vi "Objective Align.vi"() -> ()   [LabVIEW 2021]
uses:
  Objective Align Controls/Objective Align Notifier Type Def.ctl
  Objective Align Controls/Objective Align Actions.ctl
  <vilib>/vision/Image Controls.llb/IMAQ Image.ctl
  Hardware Configuration/Hardware Configuration Controls/Device Type.ctl
  Hardware Configuration/Hardware Configuration Controls/Device Function.ctl
  Device Library/Stages/Stages Controls/Stage Actions.ctl
panel:
  out "Top Z shift":dbl
  out "Bottom Z shift":dbl
  in  "Sample Z factor":dbl
  in  "Obj. Z factor":dbl
  in  "Quit":bool
  in  "Frame Accumulation":u16
  in  "CCD offset":dbl
  out "XY shift":dbl[](array[numeric])
  out "Coord":i32[][](array[numeric])
  out "Z metric":dbl[](array[numeric])
  out "ROI stack":u16[][][](array[numeric])
  in  "ROI Size":i32
  in  "XY Step Size (µm)":dbl
  in  "Pixel Size (µm)":dbl
  in  "Start Align":bool
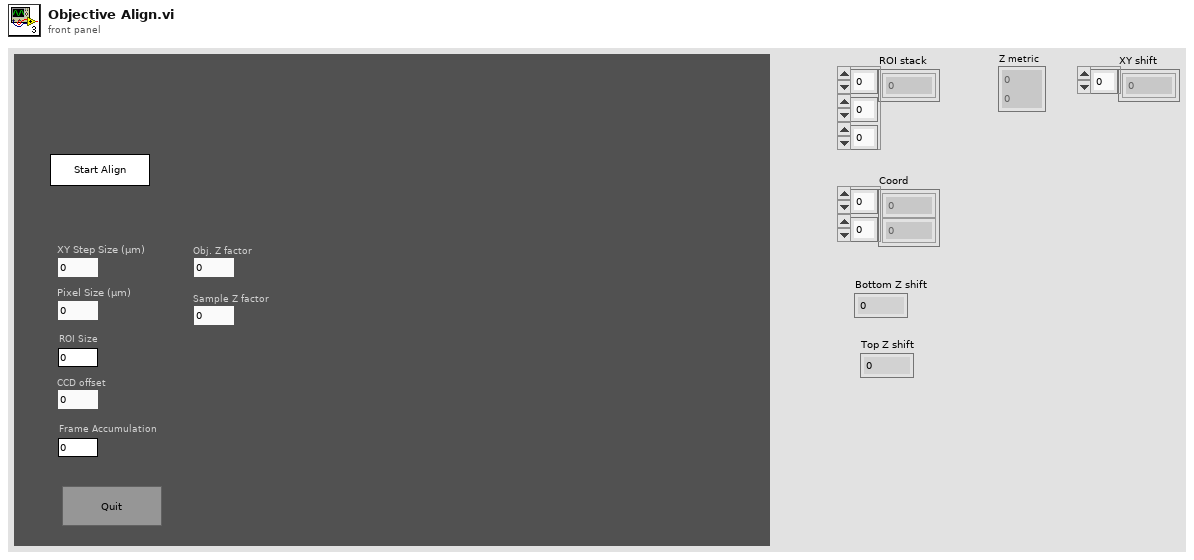
[diagram p1: front panel]
types:
  T1 = typedef "IMAQ Image.ctl" = refnum<image>
  T2 = typedef "Objective Align Actions.ctl" = enum16{"idle", "Start Align", "Move Z stage", "Move XY Stage", "Get Image", "Get Position", "Exit", "Quit"}
  T3 = typedef "Objective Align Notifier Type Def.ctl" = cluster{"Action":T2, "Pixel Size (µm)":dbl, "XY Step Size (µm)":dbl, "Image Ref":T1, "ROI Size":i32, "ROI Stack":u16[][][], "Frame Accumulation":u16, "CCD offset":dbl, "obj. Z factor":dbl, "sample Z factor ":dbl}
  T4 = typedef "Device Function.ctl" = enum16{"Primary", "Secondary", "Overview", "Wide Field Drift Correction", "642 nm Excitation", "560 nm Excitation", "940 nm Excitation", "546 nm Excitation", "488 nm Excitation", "405 nm Excitation", "Objective Drift Correction", "4Pi Focus Lock", "4Pi Objective Lock", "Objective XY", "Objective Z", "Sample XY", "Sample Coarse Z", "Sample Z", "4Pi Lower", "4Pi Upper", "Em Small", "Em Large", "Ex Small", "Ex Large", "Mojo", "Adj Cavity", "Line Scanning", "Alert"}
  T5 = typedef "Device Type.ctl" = enum16{"AOTF", "Camera", "Deformable Mirror", "Laser", "Flip Mirror", "Shutter", "Stage", "Waveform", "FPGA", "Email"}
  T6 = typedef "Stage Actions.ctl" = enum16{"Get Position", "SERVO OFF", "SERVO ON", "SERVO ON/OFF", "MVR", "MOVE", "HALT", "ONTARGET", "ERROR", "REFERENCE", "INIT", "VELOCITY", "STATUS", "EXIT", "HOME", "ZEROPOS", "NANOPOS", "ANALOG", "QUIT"}
  T7 = typedef "4Pi OBJ Lock-2D Gaussian - Best Fit Parameters.ctl" = cluster{"Amplitude":dbl, "X Position":dbl, "Y Position":dbl, "X Width":dbl, "Y Width":dbl, "Offset":dbl}
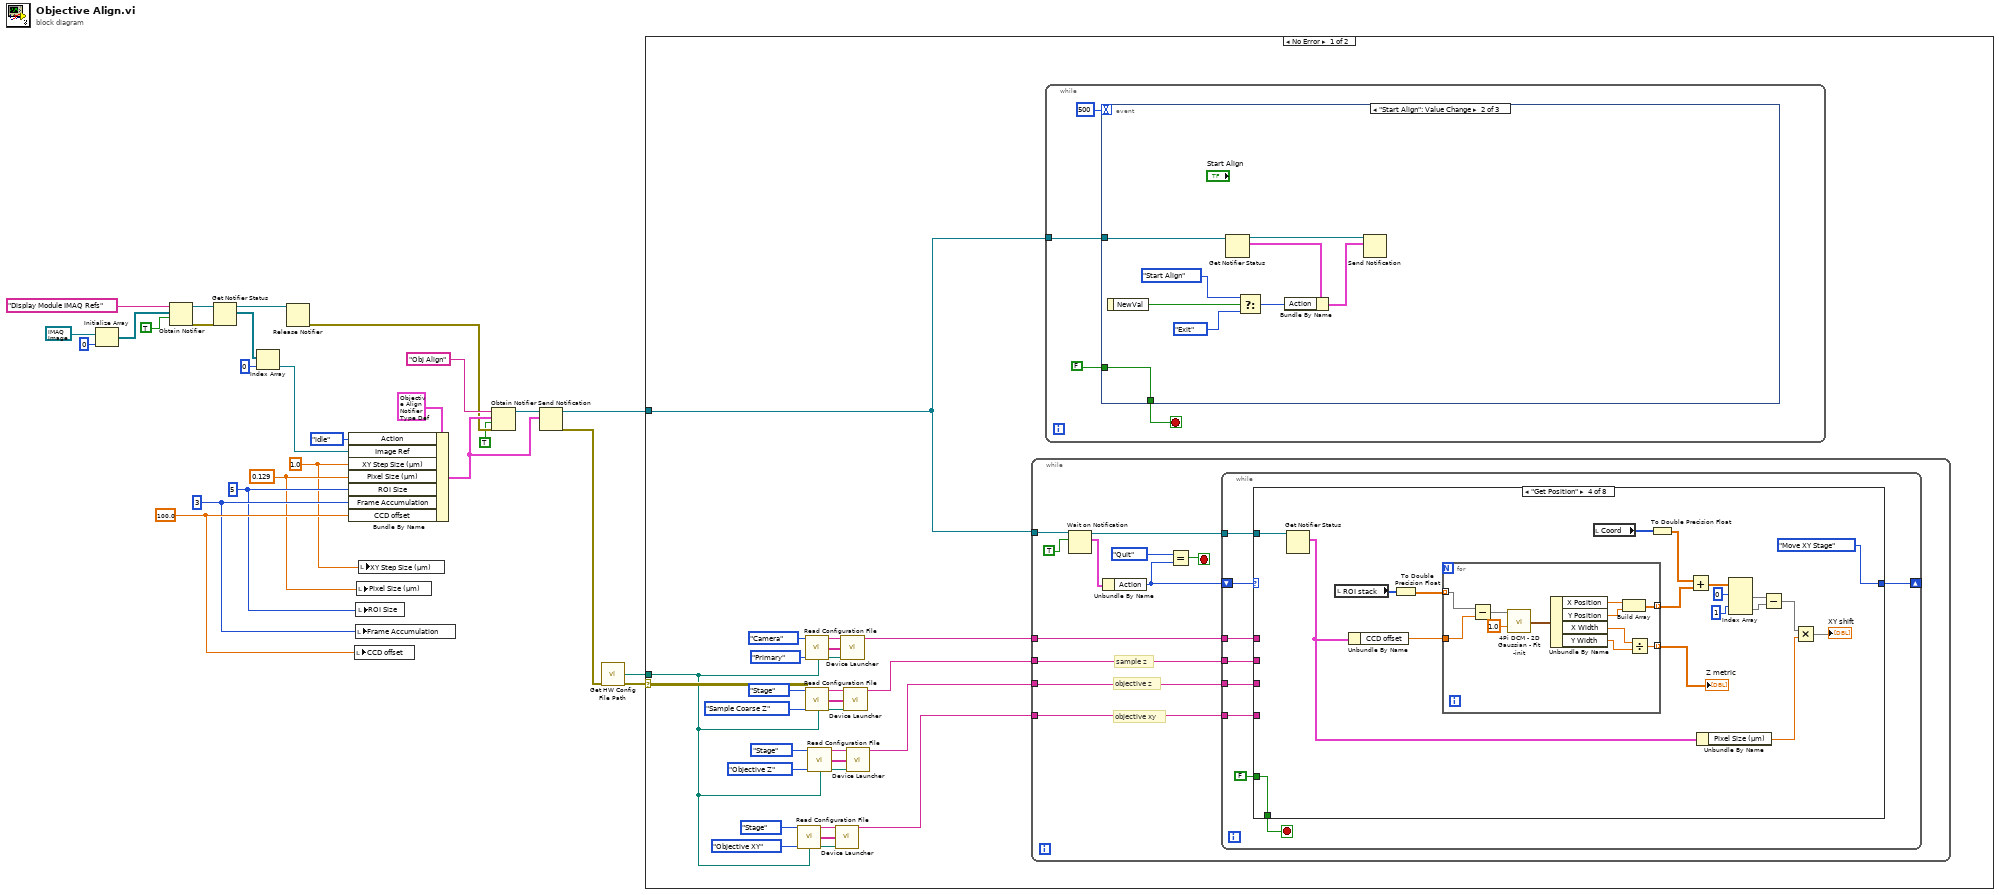
[diagram p0: block diagram]
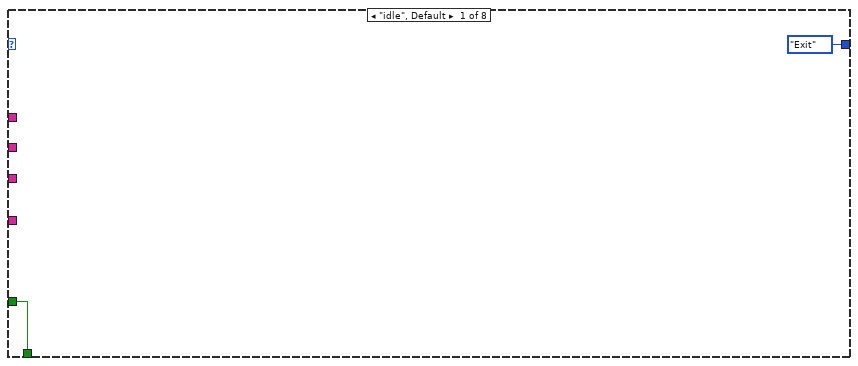
[diagram p2: hidden frame]
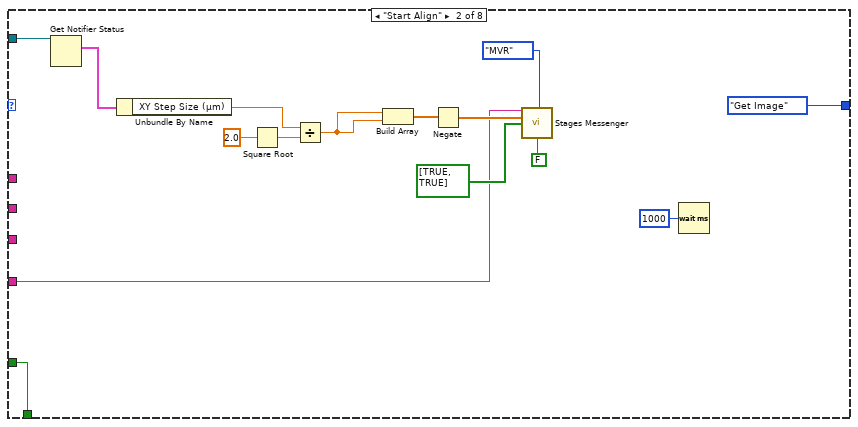
[diagram p3: hidden frame]
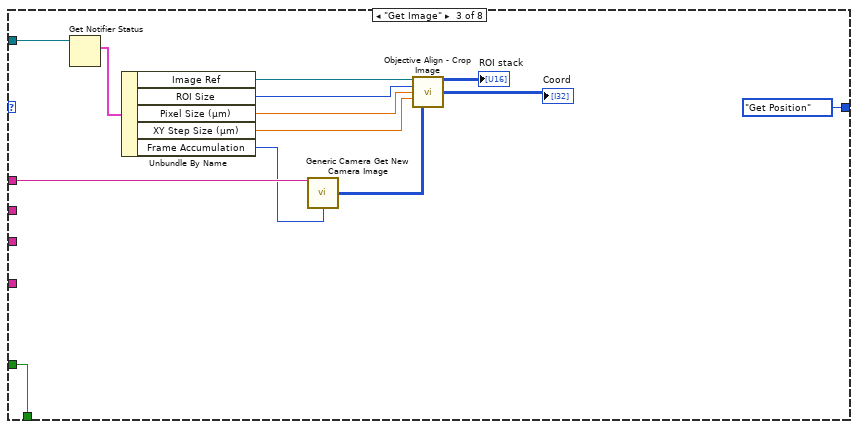
[diagram p4: hidden frame]
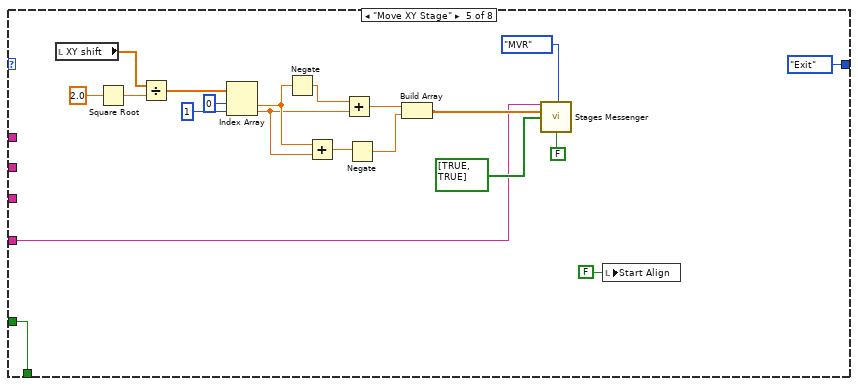
[diagram p5: hidden frame]
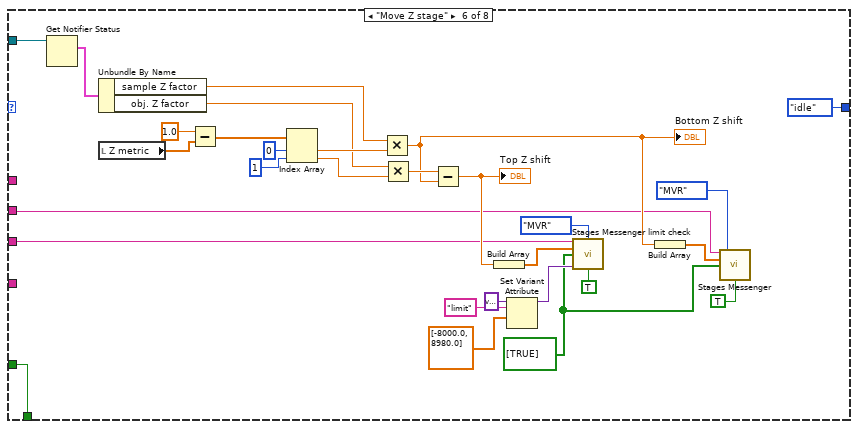
[diagram p6: hidden frame]
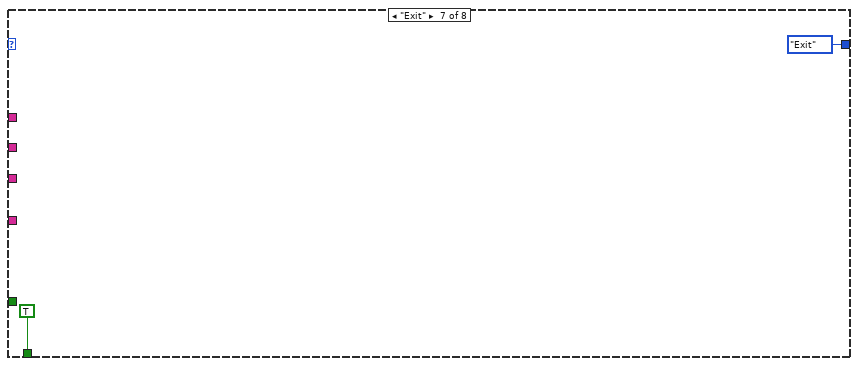
[diagram p7: hidden frame]
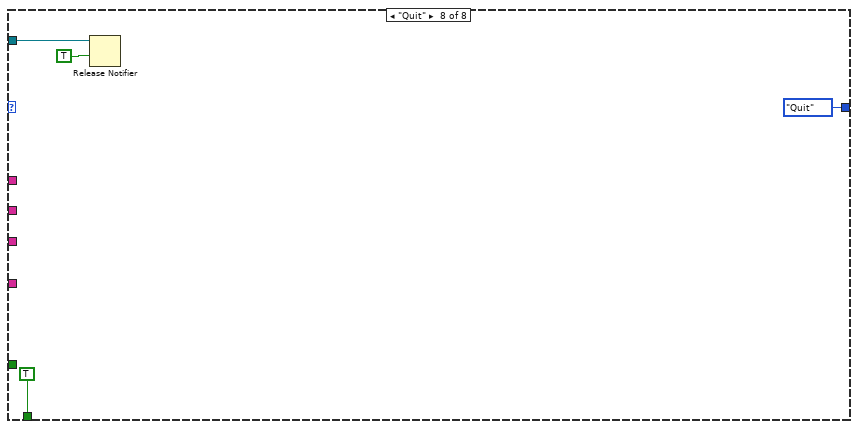
[diagram p8: hidden frame]
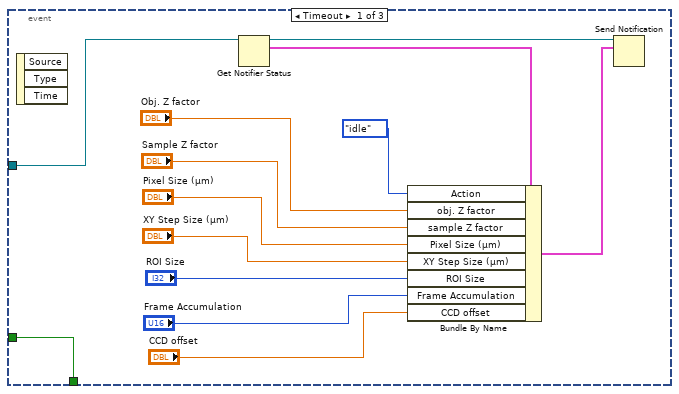
[diagram p9: hidden frame]
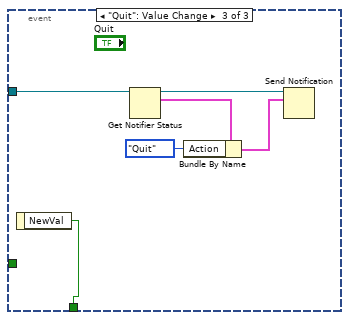
[diagram p10: hidden frame]
diagram:
  w8 = 100.0 ("CCD offset")
  w7 = u16 3 ("Frame Accumulation")
  w6 = 5 ("ROI Size")
  w5 = 0.129 ("Pixel Size (µm)")
  w4 = 1.0 ("XY Step Size (µm)")
  n1 = Initialize Array(T1 refnum ("New Image"), 0 ("dimension size")) -> (w21:T1[])
  n2 = Obtain Notifier(name (unnamed)="Display Module IMAQ Refs", notification data type=w21, create if not found? (T)=TRUE) -> (notifier out=w20:refnum<notifier>, error out=w19:errorcluster)  [unwired: 1 in, 1 out]
  n3 = Get Notifier Status(notifier=w20, error in (no error)=w19) -> (notifier out=w3:refnum<notifier>, current notification=w18:T1[])  [unwired: 3 out]
  n4 = Index Array(array=w18, index=0) -> (element=w16:T1)
  n5 = Release Notifier(notifier=w3) -> (error out=w2:errorcluster)  [unwired: 2 in, 2 out]
  n6 = Bundle By Name(cluster=T3 {"Action"=enum."Start Align", "Pixel Size (µm)"=0.0, "XY Step Size (µm)"=0.0, "Image Ref"=refnum, "ROI Size"=0, "ROI Stack"=[], "Frame Accumulation"=0, "CCD offset"=0.0, "obj. Z factor"=0.0, "sample Z factor "=0.0} ("Objective Align Notifier Type"), "Action"=Objective_Align_Actions."idle", "Image Ref"=w16, "XY Step Size (µm)"=w4, "Pixel Size (µm)"=w5, "ROI Size"=w6, "Frame Accumulation"=w7, "CCD offset"=w8) -> (w13:T3)
  n7 = local write "CCD offset"(w8) -> ()
  n8 = local write "Frame Accumulation"(w7) -> ()
  n9 = local write "ROI Size"(w6) -> ()
  n10 = local write "Pixel Size (µm)"(w5) -> ()
  n11 = local write "XY Step Size (µm)"(w4) -> ()
  n12 = Obtain Notifier(name (unnamed)="Obj Align", notification data type=w13, create if not found? (T)=TRUE, error in (no error)=w2) -> (notifier out=w14:refnum<notifier>)  [unwired: 2 out]
  n13 = Send Notification(notification=w13, notifier=w14) -> (notifier out=w9:refnum<notifier>, error out=w12:errorcluster)  [unwired: 1 in]
  n14 = call "Get HW Config File Path.vi"("Error"=w12) -> ("File Path"=w10:path, "Error"=w11:errorcluster)  [unwired: 13 in]
  n15 = case shown="No Error" w11 {
    tunnel: w9 -> [w43 _]
    tunnel: w10 -> [w29 _]
    frame No Error {
      n16 = call "Read Configuration File.vi"("Device Type"=Device_Type."Stage", "Device Function"=Device_Function."Objective XY", "Config File Path"=w29) -> ("Unique Notifier Name"=w48:string, "Device Ports/IDs/Channels"=w47:string[], "Device Engine Path"=w46:path)  [unwired: 9 in, 1 out]
      n17 = call "Read Configuration File.vi"("Device Type"=Device_Type."Camera", "Device Function"=Device_Function."Primary", "Config File Path"=w29) -> ("Unique Notifier Name"=w53:string, "Device Ports/IDs/Channels"=w51:string[], "Device Engine Path"=w52:path)  [unwired: 9 in, 1 out]
      n18 = call "Read Configuration File.vi"("Device Type"=Device_Type."Stage", "Device Function"=Device_Function."Sample Coarse Z", "Config File Path"=w29) -> ("Unique Notifier Name"=w38:string, "Device Ports/IDs/Channels"=w39:string[], "Device Engine Path"=w40:path)  [unwired: 9 in, 1 out]
      n19 = call "Read Configuration File.vi"("Device Type"=Device_Type."Stage", "Device Function"=Device_Function."Objective Z", "Config File Path"=w29) -> ("Unique Notifier Name"=w30:string, "Device Ports/IDs/Channels"=w31:string[], "Device Engine Path"=w32:path)  [unwired: 9 in, 1 out]
      n20 = call "Device Launcher.vi"("Notifier Name"=w48, "Device Ports/IDs/Channels"=w47, "Device Engine Path"=w46) -> ("Notifier Name"=w42:string)  [unwired: 11 in, 1 out]
      n21 = call "Device Launcher.vi"("Notifier Name"=w53, "Device Ports/IDs/Channels"=w51, "Device Engine Path"=w52) -> ("Notifier Name"=w41:string)  [unwired: 11 in, 1 out]
      n22 = call "Device Launcher.vi"("Notifier Name"=w38, "Device Ports/IDs/Channels"=w39, "Device Engine Path"=w40) -> ("Notifier Name"=w35:string)  [unwired: 11 in, 1 out]
      n23 = call "Device Launcher.vi"("Notifier Name"=w30, "Device Ports/IDs/Channels"=w31, "Device Engine Path"=w32) -> ("Notifier Name"=w28:string)  [unwired: 11 in, 1 out]
      n24 = while {
        tunnel: w43 -> [w62]
        tunnel: w42 -> [w57]
        tunnel: w41 -> [w56]
        tunnel: w35 -> [w55]
        tunnel: w28 -> [w54]
        stop <- w60 stop-if-true
        # "objective xy"
        # "sample z"
        # "objective z"
        n25 = Wait on Notification(notifier=w62, ignore previous (F)=TRUE) -> (notifier out=w59:refnum<notifier>, notification=w63:T3)  [unwired: 2 in, 2 out]
        n26 = Unbundle By Name(w63) -> ("Action"=w58:T2)
        n27 = Equal?(x=Objective_Align_Actions."Quit", y=w58) -> (x = y?=w60:bool)
        n28 = while {
          tunnel: w59 -> [w70]
          shift-right: [w68] -> _
          shift-left: w58 -> [w71]
          tunnel: w57 -> [w69]
          tunnel: w56 -> [w67]
          tunnel: w55 -> [w66]
          tunnel: w54 -> [w65]
          stop <- w72 stop-if-true
          n29 = case shown="\"Get Position\"" w71 {
            tunnel: FALSE -> [w74 w90 w91 w122 w135 w181 _ _]
            tunnel: [w74 w90 w91 w122 w135 w181 TRUE TRUE] -> w72
            tunnel: w70 -> [_ w89 w103 w121 _ w180 _ w187]
            tunnel: w69 -> [_ w78 _ _ w137 _ _ _]
            tunnel: [Objective_Align_Actions."Exit" ("Action") Objective_Align_Actions."Get Image" ("Action") Objective_Align_Actions."Get Position" ("Action") Objective_Align_Actions."Move XY Stage" ("Action") Objective_Align_Actions."Exit" ("Action") Objective_Align_Actions."idle" ("Action") Objective_Align_Actions."Exit" ("Action") Objective_Align_Actions."Quit" ("Action")] -> w68
            tunnel: w67 -> [_ _ w101 _ _ _ _ _]
            tunnel: w66 -> [_ _ _ _ _ w157 _ _]
            tunnel: w65 -> [_ _ _ _ _ w161 _ _]
            frame "idle", Default {
            }
            frame "Start Align" {
              n30 = Get Notifier Status(notifier=w89) -> (current notification=w88:T3)  [unwired: 1 in, 4 out]
              n31 = Unbundle By Name(w88) -> ("XY Step Size (µm)"=w85:dbl)
              n32 = Square Root(x=2.0) -> (sqrt(x)=w86:dbl)
              n33 = Divide(x=w85, y=w86) -> (x/y=w84:dbl)
              n34 = Build Array(w84, w84) -> (w83:dbl[])
              n35 = Negate(x=w83) -> (-x=w81:dbl[])
              n36 = call "Stages Messenger.vi"("Stage Notifier Name"=w78, "Actions"=Stage_Actions."MVR", "Setpoint"=w81, "Axis"=bool[] [TRUE, TRUE], "Exit While Busy?"=FALSE) -> ()  [unwired: 6 in, 5 out]
              n37 = Wait (ms)(milliseconds to wait=u32 1000) -> ()  [unwired: 1 out]
            }
            frame "Get Image" {
              n38 = Get Notifier Status(notifier=w103) -> (current notification=w102:T3)  [unwired: 1 in, 4 out]
              n39 = Unbundle By Name(w102) -> ("Image Ref"=w99:T1, "ROI Size"=w98:i32, "Pixel Size (µm)"=w97:dbl, "XY Step Size (µm)"=w96:dbl, "Frame Accumulation"=w100:u16)
              n40 = call "Generic Camera Get New Camera Image.vi"("Camera Notifier Name"=w101, "Frames"=w100) -> ("Image - U16"=w95:u16[][])  [unwired: 11 in, 2 out]
              n41 = call "Objective Align - Crop Image.vi"("Image Ref"=w99, "ROI Size"=w98, "Pixel Size (µm)"=w97, "XY Step Size (µm)"=w96, "Input Image - U16"=w95) -> ("Output Image Stack"=→"ROI stack":u16[][][], "Coord"=→"Coord":i32[][])  [unwired: 9 in]
            }
            frame "Get Position" {
              n42 = Get Notifier Status(notifier=w121) -> (current notification=w107:T3)  [unwired: 1 in, 4 out]
              n43 = local read "ROI stack"() -> (w120:u16[][][])
              n44 = Unbundle By Name(w107) -> ("CCD offset"=w118:dbl)
              n45 = To Double Precision Float(number=w120) -> (double precision float=w119:dbl[][][])
              n46 = for {
                tunnel: w119 -> [w131] mode=indexing
                tunnel: w118 -> [w130]
                tunnel: [w126] -> w117 mode=indexing
                tunnel: [w123] -> w114 mode=indexing
                n47 = Subtract(x=w131, y=w130) -> (x-y=w129:dbl[][])
                n48 = call "4Pi DCM - 2D Gaussian - Fit -init.vi"("Image In (DBL)"=w129, "width"=1.0) -> ("Best Fit Params"=w132:T7)  [unwired: 12 in, 1 out]
                n49 = Unbundle By Name(w132) -> ("X Position"=w125:dbl, "Y Position"=w124:dbl, "X Width"=w128:dbl, "Y Width"=w127:dbl)
                n50 = Build Array(w125, w124) -> (w123:dbl[])
                n51 = Divide(x=w128, y=w127) -> (x/y=w126:dbl)
              }
              "Z metric" <- w117
              n52 = local read "Coord"() -> (w116:i32[][])
              n53 = To Double Precision Float(number=w116) -> (double precision float=w115:dbl[][])
              n54 = Add(x=w115, y=w114) -> (x+y=w111:dbl[][])
              n55 = Unbundle By Name(w107) -> ("Pixel Size (µm)"=w105:dbl)
              n56 = Index Array(array=w111, index (row) #1=0 ("index"), index (row) #2=1 ("index")) -> (element #1=w110:dbl[], element #2=w109:dbl[])  [unwired: 2 in]
              n57 = Subtract(x=w110, y=w109) -> (x-y=w106:dbl[])
              n58 = Multiply(x=w106, y=w105) -> (x*y=→"XY shift":dbl[])
            }
            frame "Move XY Stage" {
              n59 = local read "XY shift"() -> (w149:dbl[])
              n60 = Square Root(x=2.0) -> (sqrt(x)=w150:dbl)
              n61 = Divide(x=w149, y=w150) -> (x/y=w148:dbl[])
              n62 = Index Array(array=w148, index #1=0 ("index"), index #2=1 ("index")) -> (element #1=w146:dbl, element #2=w145:dbl)
              n63 = Negate(x=w146) -> (-x=w147:dbl)
              n64 = Add(x=w146, y=w145) -> (x+y=w144:dbl)
              n65 = Add(x=w147, y=w145) -> (x+y=w140:dbl)
              n66 = Negate(x=w144) -> (-x=w139:dbl)
              n67 = Build Array(w140, w139) -> (w138:dbl[])
              n68 = call "Stages Messenger.vi"("Stage Notifier Name"=w137, "Actions"=Stage_Actions."MVR", "Setpoint"=w138, "Axis"=bool[] [TRUE, TRUE], "Exit While Busy?"=FALSE) -> ()  [unwired: 6 in, 5 out]
              n69 = local write "Start Align"(FALSE ("Start Align")) -> ()
            }
            frame "Move Z stage" {
              w156 = bool[] [TRUE]
              n70 = Get Notifier Status(notifier=w180) -> (current notification=w179:T3)  [unwired: 1 in, 4 out]
              n71 = Unbundle By Name(w179) -> ("sample Z factor"=w172:dbl, "obj. Z factor"=w170:dbl)
              n72 = local read "Z metric"() -> (w175:dbl[])
              n73 = Subtract(x=1.0, y=w175) -> (x-y=w174:dbl[])
              n74 = Index Array(array=w174, index #1=0 ("index"), index #2=1 ("index")) -> (element #1=w173:dbl, element #2=w171:dbl)
              n75 = Multiply(x=w172, y=w173) -> (x*y=w159:dbl)
              "Bottom Z shift" <- w159
              n76 = Multiply(x=w170, y=w171) -> (x*y=w169:dbl)
              n77 = Subtract(x=w169, y=w159) -> (x-y=w168:dbl)
              "Top Z shift" <- w168
              n78 = Build Array(w168) -> (w162:dbl[])
              n79 = Set Variant Attribute(Variant=variant ("variant"), name="limit", value=dbl[] [-8000.0, 8980.0] ("Array")) -> (Variant out=w163:variant)  [unwired: 1 in, 2 out]
              n80 = call "Stages Messenger limit check.vi"("Stage Notifier Name"=w161, "Actions"=Stage_Actions."MVR", "Setpoint"=w162, "Axis"=w156, "Misc"=w163, "Exit While Busy?"=TRUE) -> ()  [unwired: 6 in, 4 out]
              n81 = Build Array(w159) -> (w158:dbl[])
              n82 = call "Stages Messenger.vi"("Stage Notifier Name"=w157, "Actions"=Stage_Actions."MVR", "Setpoint"=w158, "Axis"=w156, "Exit While Busy?"=TRUE) -> ()  [unwired: 6 in, 5 out]
            }
            frame "Exit" {
            }
            frame "Quit" {
              n83 = Release Notifier(notifier=w187, force destroy? (F)=TRUE) -> ()  [unwired: 1 in, 3 out]
            }
          }
        }
      }
      n84 = while {
        tunnel: w43 -> [w190]
        stop <- w191 stop-if-true
        n85 = event shown="[1] \"Start Align\": Value Change" {
          selector: _ -> [_ _ _]
          dyn-events: _ -> [_ _ _]
          timeout: 500 -> [_ _ _]
          tunnel: [w205 w206 w220] -> w191
          tunnel: FALSE -> [w205 w206 _]
          tunnel: w190 -> [w204 w211 w216]
          event Timeout {
            n86 = event-data() -> ()  [unwired: 1 in, 3 out]
            n87 = Get Notifier Status(notifier=w204) -> (notifier out=w193:refnum<notifier>, current notification=w203:T3)  [unwired: 1 in, 3 out]
            n88 = Bundle By Name(cluster=w203, "Action"=Objective_Align_Actions."idle", "obj. Z factor"="Obj. Z factor", "sample Z factor"="Sample Z factor", "Pixel Size (µm)"="Pixel Size (µm)", "XY Step Size (µm)"="XY Step Size (µm)", "ROI Size"="ROI Size", "Frame Accumulation"="Frame Accumulation", "CCD offset"="CCD offset") -> (w194:T3)
            n89 = Send Notification(notification=w194, notifier=w193) -> ()  [unwired: 1 in, 2 out]
          }
          event "Start Align": Value Change {
            n90 = event-data() -> ("NewVal"=w210:bool)  [unwired: 1 in]
            n91 = Get Notifier Status(notifier=w211) -> (notifier out=w213:refnum<notifier>, current notification=w214:T3)  [unwired: 1 in, 3 out]
            n92 = Select(t=Objective_Align_Actions."Start Align" ("Action"), s=w210, f=Objective_Align_Actions."Exit") -> (s? t:f=w207:T2)
            n93 = Bundle By Name(cluster=w214, "Action"=w207) -> (w212:T3)
            n94 = Send Notification(notification=w212, notifier=w213) -> ()  [unwired: 1 in, 2 out]
          }
          event "Quit": Value Change {
            n95 = event-data() -> ("NewVal"=w220:bool)  [unwired: 1 in]
            n96 = Get Notifier Status(notifier=w216) -> (notifier out=w219:refnum<notifier>, current notification=w218:T3)  [unwired: 1 in, 3 out]
            n97 = Bundle By Name(cluster=w218, "Action"=Objective_Align_Actions."Quit") -> (w217:T3)
            n98 = Send Notification(notification=w217, notifier=w219) -> ()  [unwired: 1 in, 2 out]
          }
        }
      }
    }
    frame Error {
    }
  }
